vi "FT6301A_set load.vi"(6 "Switch Button":u16(ring) items=["off", "on"], 8 "error in (no error)":errorcluster, 9 "Load Parameter":dbl, 10 "Load Mode select":u16(ring) items=["CC mode", "CR mode", "CV mode"], 11 "VISA resource name 4":refnum<visa-resource-name>) -> (1 "error out":errorcluster)   [LabVIEW 2023]
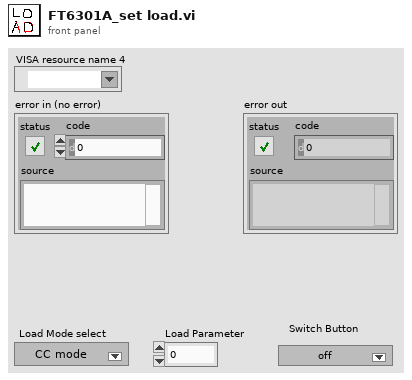
[diagram p1: front panel]
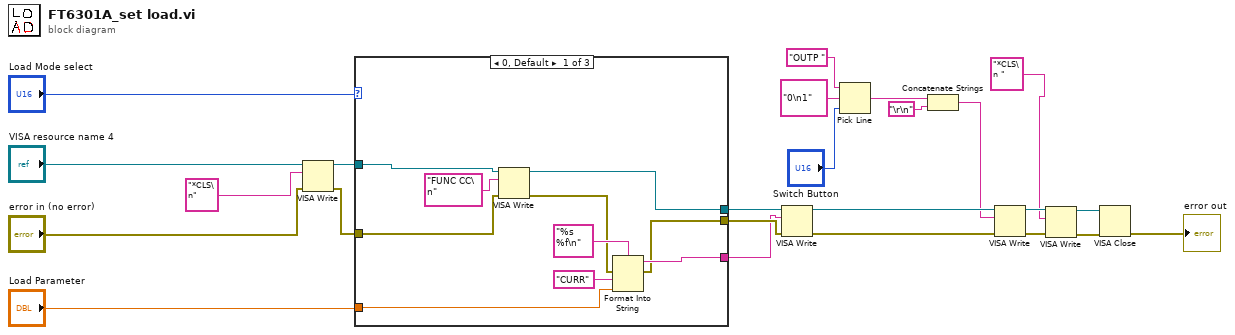
[diagram p0: block diagram]
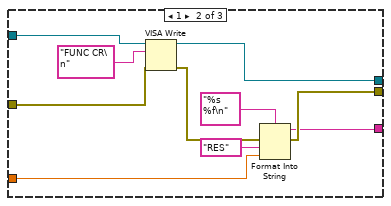
[diagram p2: hidden frame]
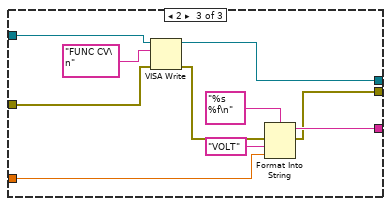
[diagram p3: hidden frame]
diagram:
  n1 = VISA Write(VISA resource name="VISA resource name 4", write buffer="*CLS\n", error in (no error)="error in (no error)") -> (VISA resource name out=w7:refnum<visa-resource-name>, error out=w8:errorcluster)  [unwired: 1 out]
  n2 = case shown="0, Default" "Load Mode select" {
    tunnel: "Load Parameter" -> [w29 w40 w50]
    tunnel: w8 -> [w30 w39 w51]
    tunnel: [w31 w37 w48] -> w13
    tunnel: [w25 w36 w46] -> w12
    tunnel: [w28 w35 w49] -> w11
    tunnel: w7 -> [w27 w38 w52]
    frame 0, Default {
      n3 = VISA Write(VISA resource name=w27, write buffer="FUNC CC\n", error in (no error)=w30) -> (VISA resource name out=w31:refnum<visa-resource-name>, error out=w26:errorcluster)  [unwired: 1 out]
      n4 = Format Into String(format string="%s %f\n", error in=w26, "CURR" ("write buffer"), w29) -> (resulting string=w28:string, error out=w25:errorcluster)  [unwired: 1 in]
    }
    frame 1 {
      n5 = VISA Write(VISA resource name=w38, write buffer="FUNC CR\n", error in (no error)=w39) -> (VISA resource name out=w37:refnum<visa-resource-name>, error out=w42:errorcluster)  [unwired: 1 out]
      n6 = Format Into String(format string="%s %f\n", error in=w42, "RES" ("write buffer"), w40) -> (resulting string=w35:string, error out=w36:errorcluster)  [unwired: 1 in]
    }
    frame 2 {
      n7 = VISA Write(VISA resource name=w52, write buffer="FUNC CV\n", error in (no error)=w51) -> (VISA resource name out=w48:refnum<visa-resource-name>, error out=w47:errorcluster)  [unwired: 1 out]
      n8 = Format Into String(format string="%s %f\n", error in=w47, "VOLT" ("write buffer"), w50) -> (resulting string=w49:string, error out=w46:errorcluster)  [unwired: 1 in]
    }
  }
  n9 = VISA Write(VISA resource name=w13, write buffer=w11, error in (no error)=w12) -> (VISA resource name out=w22:refnum<visa-resource-name>, error out=w21:errorcluster)  [unwired: 1 out]
  n10 = Pick Line(string ("")="OUTP ", multi-line string="0\n1" ("string (\"\")"), line index="Switch Button") -> (output string=w17:string)
  n11 = Concatenate Strings(w17, "\r\n") -> (w16:string)
  n12 = VISA Write(VISA resource name=w22, write buffer=w16, error in (no error)=w21) -> (VISA resource name out=w5:refnum<visa-resource-name>, error out=w3:errorcluster)  [unwired: 1 out]
  n13 = VISA Write(VISA resource name=w5, write buffer="*CLS\n " ("string (\"\")"), error in (no error)=w3) -> (VISA resource name out=w4:refnum<visa-resource-name>, error out=w2:errorcluster)  [unwired: 1 out]
  n14 = VISA Close(VISA resource name=w4, error in (no error)=w2) -> (error out=→"error out":errorcluster)
